vi "1C.1 SmallRCSense.vi"(10 "Wind Direction":T3 format="%05.1f", 11 "Wind Speed":dbl) -> (0 "Apparent Wind\nSpeed":T1, 1 "Apparent Wind\nDirection":T2, 2 "Boat\nVelocity":T4, 3 "Heading":T3 format="%05.1f", 4 "Eye in the Sky":T6(plugin-control), 5 "Boat Location":T5)   [LabVIEW 2011]
doc: "TODO: finish camera interpreter\nTODO: arrange this to be easier to convert for future boats!"
uses:
  2-RIO/2 Typedefs/UTM Location.ctl
  2-RIO/2 Typedefs/Velocity.ctl
  2-RIO/2 Typedefs/heading.ctl
  2-RIO/2 Typedefs/apparent wind direction.ctl
  2-RIO/2 Typedefs/apparent wind speed.ctl
  2-RIO/2 Globals/2 Global.vi
panel:
  out "Frame Rate":dbl
  out "Apparent Wind\nin global ref frame":T4
  out "Absolute Wind":T4
  in  "Add Randomness\nTo Wind Measurement":bool
  # "UNFINISHED\nTODO: finish camera interpreter, and test"
  # "(in boat ref frame)"
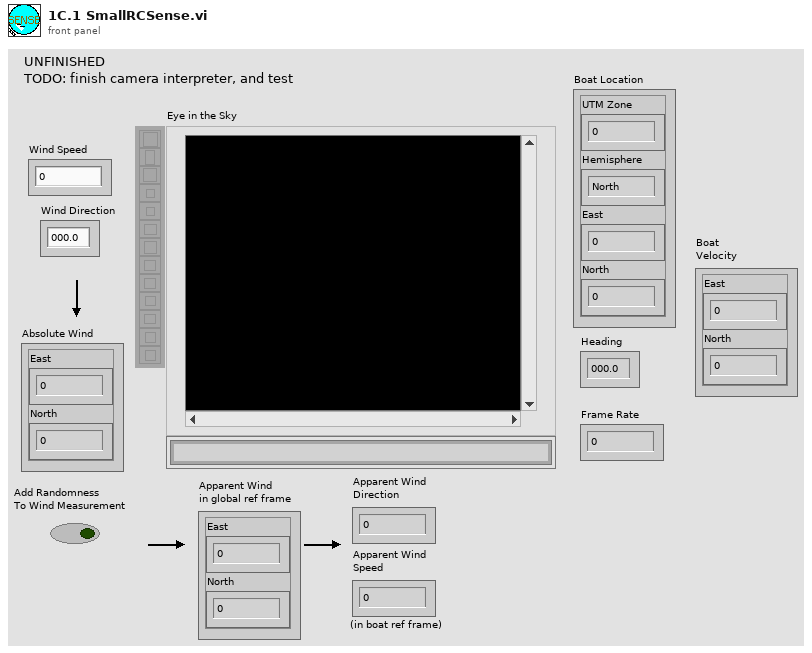
[diagram p1: front panel]
types:
  T1 = typedef "apparent wind speed.ctl" = dbl
  T2 = typedef "apparent wind direction.ctl" = dbl
  T3 = typedef "heading.ctl" = dbl
  T4 = typedef "Velocity.ctl" = cluster{"East":dbl, "North":dbl}
  T5 = typedef "UTM Location.ctl" = cluster{"UTM Zone":dbl, "Hemisphere":enum16{"North", "South"}, "East":dbl, "North":dbl}
  T6 = typedef "IMAQ Image.ctl" = refnum<image>
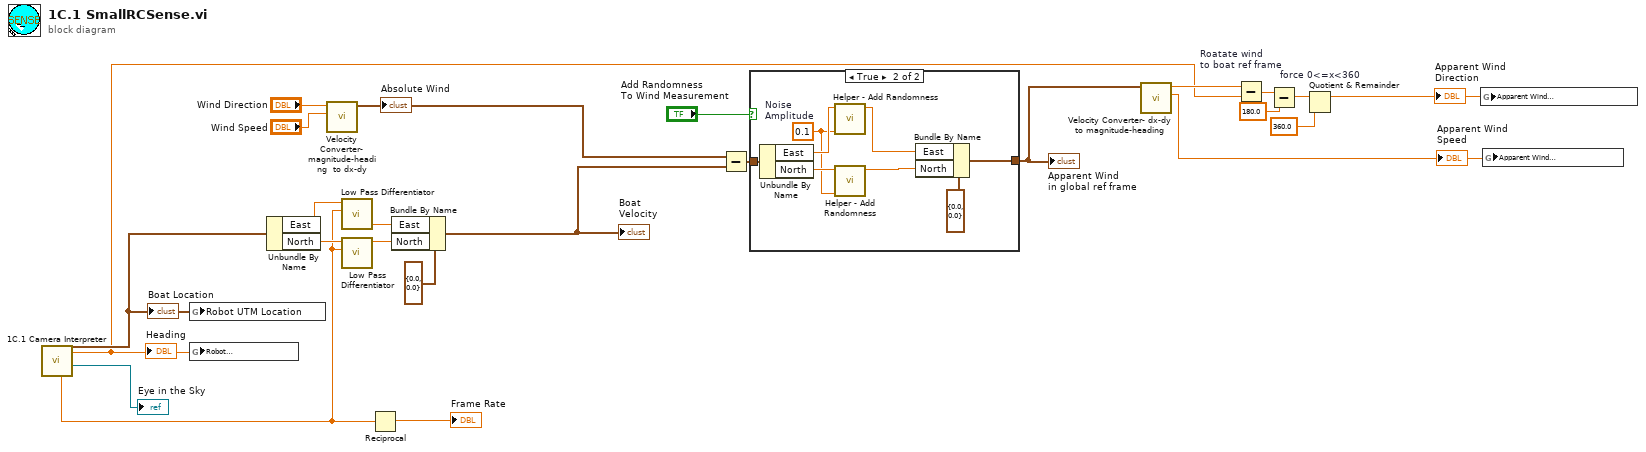
[diagram p0: block diagram]
diagram:
  n1 = call "1C.1 Camera Interpreter.vi"() -> ("Overhead Image"=→"Eye in the Sky":T6, "Heading"=w2:T3, "Boat Location"=w3:T5, "Time Elapsed (s)\nSince Last Image"=w12:dbl)  [unwired: 7 in, 1 out]
  "Boat Location" <- w3
  "Heading" <- w2
  n2 = global write "2 Global.vi" "Robot UTM Location"(w3) -> ()
  n3 = global write "2 Global.vi" "Robot\nHeading"(w2) -> ()
  n4 = Unbundle By Name(w3) -> ("East"=w23:dbl, "North"=w22:dbl)
  n5 = call "Velocity Converter- magnitude-heading  to dx-dy.vi"("Magnitude"="Wind Speed", "Heading"="Wind Direction") -> ("Vector Out"=w15:T4)  [unwired: 9 in]
  "Absolute Wind" <- w15
  n6 = call "Low Pass Differentiator.vi"("dt"=w12, "X"=w23) -> ("dX, smoothed"=w20:dbl)  [unwired: 9 in]
  n7 = call "Low Pass Differentiator.vi"("dt"=w12, "X"=w22) -> ("dX, smoothed"=w21:dbl)  [unwired: 9 in]
  n8 = Reciprocal(x=w12) -> (1/x=→"Frame Rate":dbl)
  n9 = Bundle By Name(cluster=T4 {"East"=0.0, "North"=0.0} ("Velocity 2"), "East"=w20, "North"=w21) -> (w1:T4)
  "Boat\nVelocity" <- w1
  n10 = Subtract(x=w15, y=w1) -> (x-y=w19:T4)
  n11 = case shown="True" "Add Randomness\nTo Wind Measurement" {
    tunnel: [w25 w33] -> w6
    tunnel: w19 -> [w25 w32]
    frame False {
    }
    frame True {
      w27 = 0.1  # Noise Amplitude
      n12 = Unbundle By Name(w32) -> ("East"=w31:dbl, "North"=w30:dbl)
      n13 = call "Helper - Add Randomness.vi"("Amplitude\n(default 1)"=w27, "Numeric in"=w31) -> ("Numeric out"=w28:dbl)  [unwired: 9 in]
      n14 = call "Helper - Add Randomness.vi"("Amplitude\n(default 1)"=w27, "Numeric in"=w30) -> ("Numeric out"=w29:dbl)  [unwired: 9 in]
      n15 = Bundle By Name(cluster=T4 {"East"=0.0, "North"=0.0} ("Apparent Wind 2"), "East"=w28, "North"=w29) -> (w33:T4)
    }
  }
  "Apparent Wind\nin global ref frame" <- w6
  n16 = call "Velocity Converter- dx-dy to magnitude-heading.vi"("Vector In"=w6) -> ("Magnitude Out"=w4:dbl, "Heading Out"=w9:T3)  [unwired: 9 in]
  "Apparent Wind\nSpeed" <- w4
  n17 = Subtract "Roatate wind\nto boat ref frame"(x=w9, y=w2) -> (x-y=w11:T3)
  n18 = Subtract(x=w11, y=T3 180.0) -> (x-y=w8:T3)
  n19 = Quotient & Remainder "force 0<=x<360"(x=w8, y=T3 360.0) -> (x-y*floor(x/y)=w5:T3)  [unwired: 1 out]
  "Apparent Wind\nDirection" <- w5
  n20 = global write "2 Global.vi" "Apparent Wind\nDirection"(w5) -> ()
  n21 = global write "2 Global.vi" "Apparent Wind\nSpeed"(w4) -> ()
